vi "CheckZero.vi"(10 "FrameNumIn":dbl, 11 "Markers Coords":dbl[][](array[numeric])) -> (0 "FrameNumOut":dbl, 2 "Pelvis Markers":dbl[](array[numeric]), 3 "trunk markers":dbl[](array[numeric]))   [LabVIEW 2017]
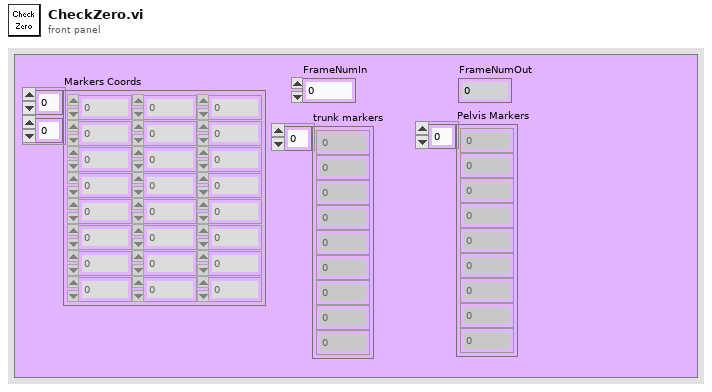
[diagram p1: front panel]
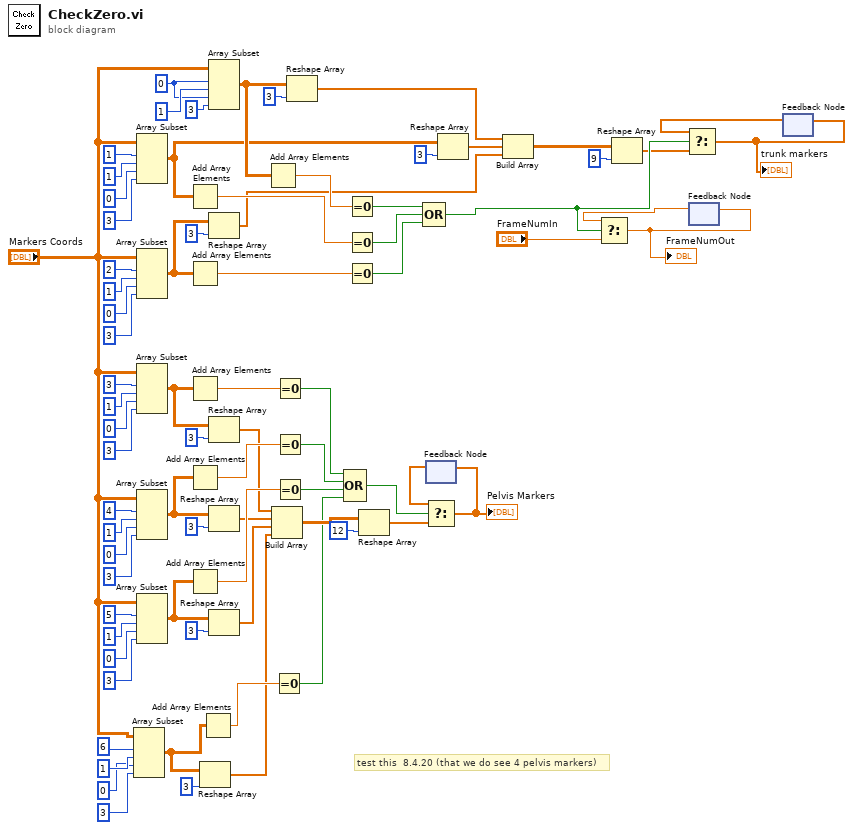
[diagram p0: block diagram]
diagram:
  w76 = 0 ("index")
  # "test this  8.4.20 (that we do see 4 pelvis markers)"
  n1 = Array Subset(array="Markers Coords", index (row)=6 ("index"), length (row)=1 ("length"), index (col)=0 ("index"), length (col)=3 ("length")) -> (w4:dbl[][])
  n2 = Array Subset(array="Markers Coords", index (row)=1 ("index"), length (row)=1 ("length"), index (col)=0 ("index"), length (col)=3 ("length")) -> (w21:dbl[][])
  n3 = Array Subset(array="Markers Coords", index (row)=2 ("index"), length (row)=1 ("length"), index (col)=0 ("index"), length (col)=3 ("length")) -> (w20:dbl[][])
  n4 = Array Subset(array="Markers Coords", index (row)=3 ("index"), length (row)=1 ("length"), index (col)=0 ("index"), length (col)=3 ("length")) -> (w32:dbl[][])
  n5 = Array Subset(array="Markers Coords", index (row)=4 ("index"), length (row)=1 ("length"), index (col)=0 ("index"), length (col)=3 ("length")) -> (w29:dbl[][])
  n6 = Array Subset(array="Markers Coords", index (row)=5 ("index"), length (row)=1 ("length"), index (col)=0 ("index"), length (col)=3 ("length")) -> (w34:dbl[][])
  n7 = Add Array Elements(numeric array=w21) -> (sum=w68:dbl)
  n8 = Add Array Elements(numeric array=w20) -> (sum=w67:dbl)
  n9 = Add Array Elements(numeric array=w32) -> (sum=w47:dbl)
  n10 = Add Array Elements(numeric array=w29) -> (sum=w46:dbl)
  n11 = Add Array Elements(numeric array=w34) -> (sum=w45:dbl)
  n12 = Reshape Array(w4, 3 ("dimension size")) -> (w2:dbl[])
  n13 = Add Array Elements(numeric array=w4) -> (sum=w3:dbl)
  n14 = Array Subset(array="Markers Coords", index (row)=w76, length (row)=1 ("length"), index (col)=w76, length (col)=3 ("length")) -> (w22:dbl[][])
  n15 = Reshape Array(w20, 3 ("dimension size")) -> (w17:dbl[])
  n16 = Reshape Array(w32, 3 ("dimension size")) -> (w26:dbl[])
  n17 = Reshape Array(w29, 3 ("dimension size")) -> (w27:dbl[])
  n18 = Reshape Array(w34, 3 ("dimension size")) -> (w28:dbl[])
  n19 = Add Array Elements(numeric array=w22) -> (sum=w69:dbl)
  n20 = Build Array(w26, w27, w28, w2) -> (w25:dbl[][])
  n21 = Equal To 0?(x=w3) -> (x = 0?=w1:bool)
  n22 = Equal To 0?(x=w47) -> (x = 0?=w44:bool)
  n23 = Equal To 0?(x=w46) -> (x = 0?=w43:bool)
  n24 = Equal To 0?(x=w45) -> (x = 0?=w42:bool)
  n25 = Reshape Array(w22, 3 ("dimension size")) -> (w19:dbl[])
  n26 = Compound Arithmetic op=OR(w44, w43, w42, w1) -> (w38:bool)
  n27 = Equal To 0?(x=w69) -> (x = 0?=w66:bool)
  n28 = Equal To 0?(x=w68) -> (x = 0?=w65:bool)
  n29 = Equal To 0?(x=w67) -> (x = 0?=w64:bool)
  n30 = Reshape Array(w25, 12 ("dimension size")) -> (w23:dbl[])
  n31 = Compound Arithmetic op=OR(w66, w65, w64) -> (w57:bool)
  n32 = feedback #1() -> (w36:dbl[])  [unwired: 1 in]
  n33 = Select(t=w36, s=w38, f=w23) -> (s? t:f=w37:dbl[])
  "Pelvis Markers" <- w37
  n34 = feedback-in #1(w37) -> ()
  n35 = Reshape Array(w21, 3 ("dimension size")) -> (w18:dbl[])
  n36 = Build Array(w19, w18, w17) -> (w16:dbl[][])
  n37 = Reshape Array(w16, 9 ("dimension size")) -> (w11:dbl[])
  n38 = feedback #2() -> (w58:dbl)  [unwired: 1 in]
  n39 = Select(t=w58, s=w57, f="FrameNumIn") -> (s? t:f=w59:dbl)
  "FrameNumOut" <- w59
  n40 = feedback-in #2(w59) -> ()
  n41 = feedback #3() -> (w63:dbl[])  [unwired: 1 in]
  n42 = Select(t=w63, s=w57, f=w11) -> (s? t:f=w35:dbl[])
  "trunk markers" <- w35
  n43 = feedback-in #3(w35) -> ()
